vi "Class_Find Children.vi"(0 "(DCmd) in":refnum<class>) -> (2 "CMD Array":refnum<class>[](array[class]), 3 "Name Array":string[](array[string]))   [LabVIEW 2015]
panel:
  out "size(s) 2":i32
  out "size(s)":i32
  out "Last Class":path
  out "error in 2":errorcluster
  in  "error in":errorcluster
  out "Source folder":path
  out "class path":path
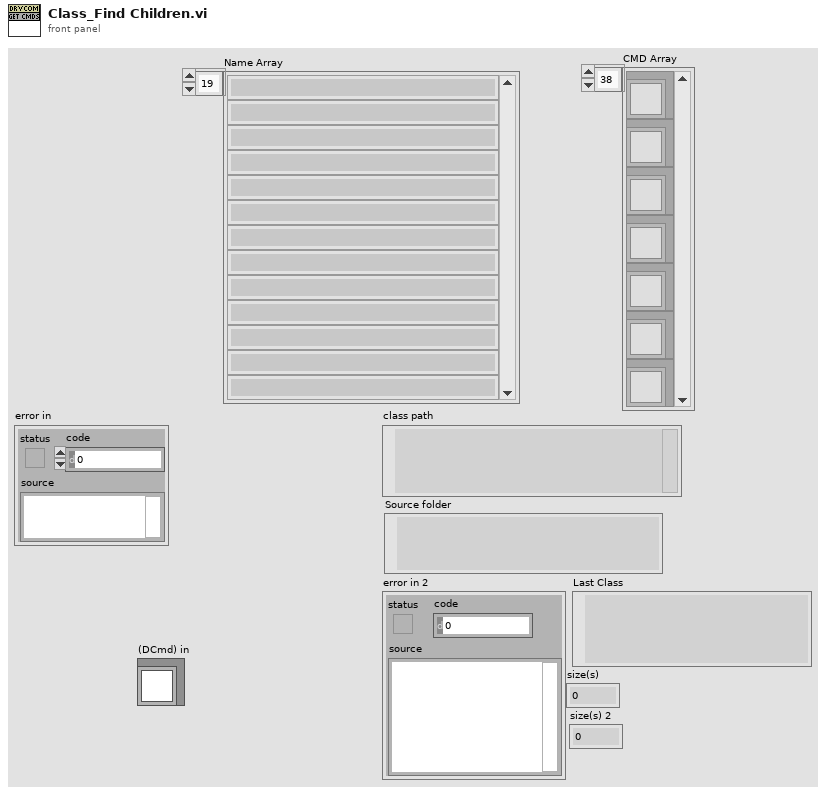
[diagram p1: front panel]
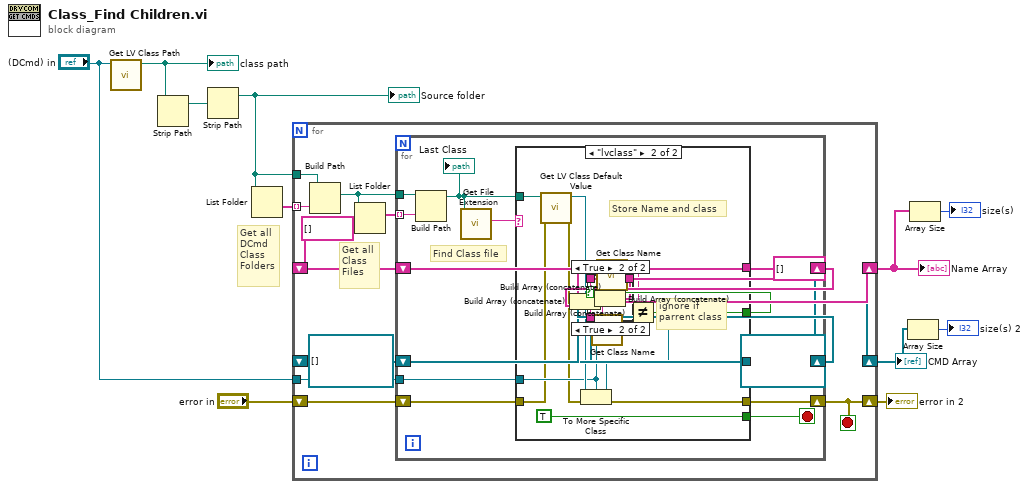
[diagram p0: block diagram]
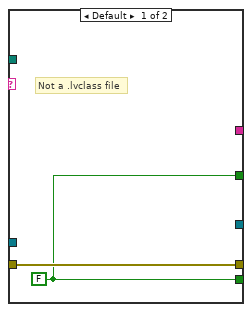
[diagram p4: hidden frame]
diagram:
  # "Get all \nDCmd\nClass\nFolders"
  n1 = call <vilib>:"Get LV Class Path.vi"("object"="(DCmd) in") -> ("class path"=w13:path)  [unwired: 9 in, 1 out]
  "class path" <- w13
  n2 = Strip Path(path=w13) -> (stripped path=w12:path)  [unwired: 1 out]
  n3 = Strip Path(path=w12) -> (stripped path=w10:path)  [unwired: 1 out]
  "Source folder" <- w10
  n4 = List Folder(path=w10) -> (folder names=w11:string[])  [unwired: 3 in, 3 out]
  n5 = for {
    tunnel: w11 -> [w27] mode=indexing
    tunnel: w10 -> [w28]
    tunnel: "(DCmd) in" -> [w24]
    shift-right: [w22] -> w7
    shift-left: "error in" -> [w23]
    shift-right: [w18] -> w4
    shift-left: string[] [] -> [w19]
    shift-right: [w16] -> w3
    shift-left: refnum<class>[] [] -> [w17]
    stop <- w22 stop-if-true
    # "Get all \nClass\nFiles"
    n6 = Build Path(base path=w28, name or relative path=w27) -> (appended path=w25:path)
    n7 = List Folder(path=w25) -> (filenames=w26:string[])  [unwired: 3 in, 3 out]
    n8 = for {
      tunnel: w26 -> [w43] mode=indexing
      tunnel: w25 -> [w42]
      tunnel: w24 -> [w39]
      shift-right: [w36] -> w22
      shift-left: w23 -> [w37]
      shift-right: [w31] -> w21
      shift-left: string[] [] ("Array") -> [w32]
      shift-right: [w29] -> w20
      shift-left: refnum<class>[] [] ("Array") -> [w30]
      stop <- w38 stop-if-true
      # "Find Class file"
      n9 = Build Path(base path=w42, name or relative path=w43) -> (appended path=w40:path)
      "Last Class" <- w40
      n10 = call <vilib>:"Get File Extension.vi"("file"=w40) -> ("lowercase file extension"=w41:string)  [unwired: 6 in, 4 out]
      n11 = case shown="\"lvclass\"" w41 {
        tunnel: w40 -> [_ w64]
        tunnel: w39 -> [_ w60]
        tunnel: [_ w55] -> w34
        tunnel: [w52 TRUE] -> w38
        tunnel: w37 -> [w53 w58]
        tunnel: [w53 w62] -> w36
        tunnel: [_ w56] -> w35
        tunnel: [w52 w54] -> w33
        frame Default {
          w52 = FALSE
          # "Not a .lvclass file"
        }
        frame "lvclass" {
          # "Store Name and class"
          # "ignore if \nparrent class"
          n12 = call <vilib>:"Get LV Class Default Value.vi"("error in (no error)"=w58, "class path"=w64) -> ("error out"=w57:errorcluster, "object"=w61:refnum<class>)  [unwired: 8 in]
          n13 = To More Specific Class(target class=w60, reference=w61, error in=w57) -> (specific class reference=w55:refnum<class>, error out=w62:errorcluster)
          n14 = call "Get Class Name.vi"("lvclass"=w60) -> ("Child Name"=w59:string)  [unwired: 3 in, 1 out]
          n15 = call "Get Class Name.vi"("lvclass"=w61) -> ("Child Name"=w56:string)  [unwired: 3 in, 1 out]
          n16 = Not Equal?(x=w56, y=w59) -> (x != y?=w54:bool)
        }
      }
      n17 = case shown="True" w33 {
        tunnel: w30 -> [w44 w46]
        tunnel: w34 -> [_ w45]
        tunnel: [w44 w47] -> w29
        frame False {
        }
        frame True {
          n18 = Build Array (concatenate)(w46, w45) -> (w47:refnum<class>[])
        }
      }
      n19 = case shown="True" w33 {
        tunnel: w32 -> [w48 w50]
        tunnel: w35 -> [_ w49]
        tunnel: [w48 w51] -> w31
        frame False {
        }
        frame True {
          n20 = Build Array (concatenate)(w50, w49) -> (w51:string[])
        }
      }
    }
    n21 = Build Array (concatenate)(w17, w20) -> (w16:refnum<class>[])
    n22 = Build Array (concatenate)(w19, w21) -> (w18:string[])
  }
  "CMD Array" <- w3
  "error in 2" <- w7
  "Name Array" <- w4
  n23 = Array Size(array=w3) -> (size(s)=→"size(s) 2":i32)
  n24 = Array Size(array=w4) -> (size(s)=→"size(s)":i32)
